vi "sv_Scale Swept Measurements to EU.vi"(4 "response(s) settings.response":T4(array[cluster]) {"channel info"."pregain" format="%.2f"; "channel info"."weighting filter" items=["Linear", "A-weighting", "B-weighting", "C-weighting", "ITU-R 468-4", "Dolby", "CCITT", "C-message", "Wb", "Wc", "Wd", "We", "Wf", "Wh", "Wj", "Wk", "Wm", "AES17 20 kHz lowpass", "AES17 40 kHz lowpass", "AES17 20 kHz highpass", "AES17 40 kHz highpass"]; "channel info"."dB reference" format="%^.1e"; "channel info"."engineering units" items=["custom..."=0, "V"=1, "A"=21, "C"=30, "pC"=31, "s"=32, "-"=29, "Pa"=2, "N"=20, "g"=3, "m/s^2"=4, "m/s"=5, "m"=6, "mm/s"=12, "mm"=13, "micron/s"=14, "micron"=15, "in/s^2"=7, "in/s"=8, "in"=9, "mil/s"=10, "mil"=11, "rad/s^2"=16, "rad/s"=17, "rad"=18, "deg/s^2"=26, "deg/s"=27, "deg"=28, "RPM"=22, "cycle/s^2"=23, "Hz"=24, "cycle"=25, "strain"=19]; "channel info"."sensor sensitivity" format="%#_5f"}, 6 "stimulus settings.stimulus":T5(array[cluster]) {"channel info"."pregain" format="%.2f"; "channel info"."weighting filter" items=["Linear", "A-weighting", "B-weighting", "C-weighting", "ITU-R 468-4", "Dolby", "CCITT", "C-message", "Wb", "Wc", "Wd", "We", "Wf", "Wh", "Wj", "Wk", "Wm", "AES17 20 kHz lowpass", "AES17 40 kHz lowpass", "AES17 20 kHz highpass", "AES17 40 kHz highpass"]; "channel info"."dB reference" format="%^.1e"; "channel info"."engineering units" items=["custom..."=0, "V"=1, "A"=21, "C"=30, "pC"=31, "s"=32, "-"=29, "Pa"=2, "N"=20, "g"=3, "m/s^2"=4, "m/s"=5, "m"=6, "mm/s"=12, "mm"=13, "micron/s"=14, "micron"=15, "in/s^2"=7, "in/s"=8, "in"=9, "mil/s"=10, "mil"=11, "rad/s^2"=16, "rad/s"=17, "rad"=18, "deg/s^2"=26, "deg/s"=27, "deg"=28, "RPM"=22, "cycle/s^2"=23, "Hz"=24, "cycle"=25, "strain"=19]; "channel info"."sensor sensitivity" format="%#_5f"}, 7 "unscaled response magnitude in":dbl format="%.2f", 8 "unscaled measurements":T6 {"harmonic components [ratio]" format="%.2f"; "THD [ratio]" format="%.2f"; "FRF Measurements"."Im [response]" format="%.2f"; "FRF Measurements"."Re [response]" format="%.2f"; "FRF Measurements"."Im [stimulus]" format="%.2f"; "FRF Measurements"."Re [stimulus]" format="%.2f"; "RMS response" format="%.2f"; "RMS stimulus" format="%.2f"}) -> (0 "scaled measurements":T6 {"harmonic components [ratio]" format="%.2f"; "THD [ratio]" format="%.2f"; "FRF Measurements"."Im [response]" format="%.2f"; "FRF Measurements"."Re [response]" format="%.2f"; "FRF Measurements"."Im [stimulus]" format="%.2f"; "FRF Measurements"."Re [stimulus]" format="%.2f"; "RMS response" format="%.2f"; "RMS stimulus" format="%.2f"}, 5 "unscaled response magnitude out":dbl format="%.2f")   [LabVIEW 2017, in "SoundVib_SweptSine.lvlib"]
uses:
  <vilib>/addons/Sound and Vibration/svt_Swept Sine/SoundVib_SweptSine.lvlib
  <vilib>/addons/_NISVFA/_Shared subVIs/Controls/svc_Channel Info.ctl
  <vilib>/addons/_NISVFA/_Shared subVIs/Controls/svc_Engineering Units Text Ring.ctl
  <vilib>/addons/_NISVFA/_Shared subVIs/Controls/svc_Weighting Filter Text Ring.ctl
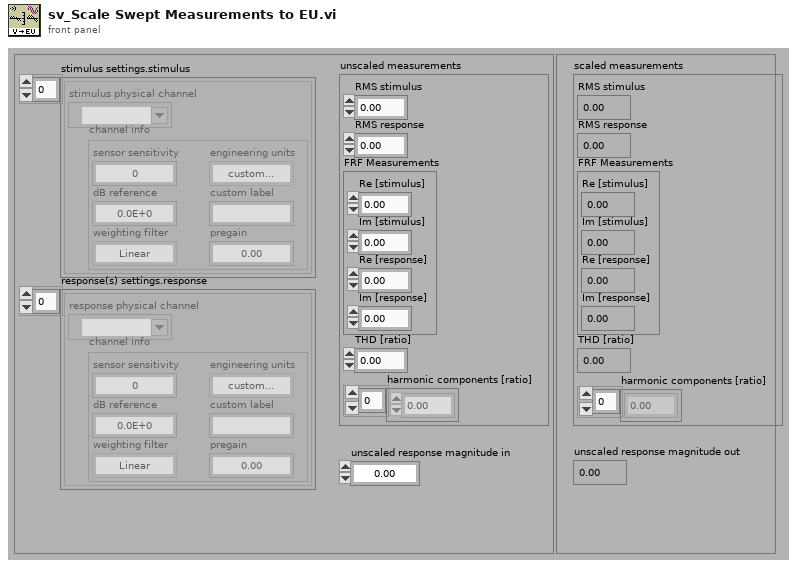
[diagram p1: front panel]
types:
  T1 = typedef "svc_Channel Info.ctl" = cluster{"sensor sensitivity":dbl, "engineering units":T2, "dB reference":dbl, "custom label":string, "weighting filter":T3, "pregain":dbl}
  T2 = typedef "svc_Engineering Units Text Ring.ctl" = u16
  T3 = typedef "svc_Weighting Filter Text Ring.ctl" = u16
  T4 = cluster{"response physical channel":tag, "channel info":T1}[]
  T5 = cluster{"stimulus physical channel":tag, "channel info":T1}[]
  T6 = cluster{"RMS stimulus":dbl, "RMS response":dbl, "FRF Measurements":cluster{"Re [stimulus]":dbl, "Im [stimulus]":dbl, "Re [response]":dbl, "Im [response]":dbl}, "THD [ratio]":dbl, "harmonic components [ratio]":dbl[]}
  T7 = cluster{"Re [stimulus]":dbl, "Im [stimulus]":dbl, "Re [response]":dbl, "Im [response]":dbl}
  T8 = cluster{"stimulus physical channel":tag, "channel info":T1}
  T9 = cluster{"response physical channel":tag, "channel info":T1}
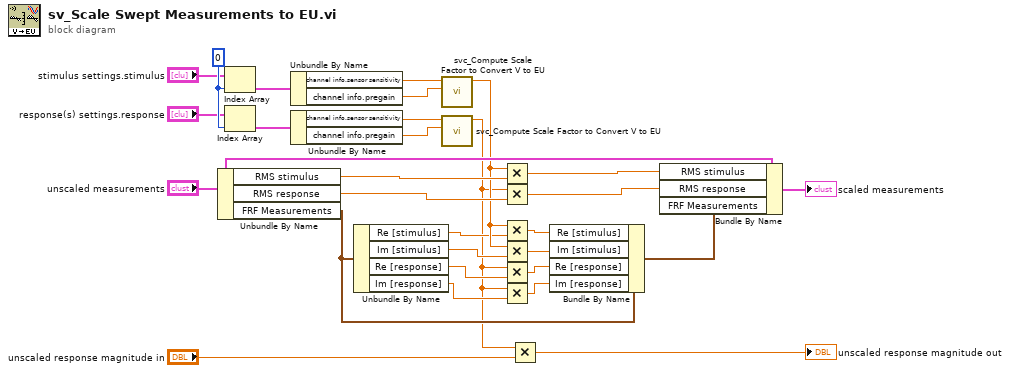
[diagram p0: block diagram]
diagram:
  w10 = 0 ("index")
  n1 = Unbundle By Name("unscaled measurements") -> ("RMS stimulus"=w17:dbl, "RMS response"=w16:dbl, "FRF Measurements"=w21:T7)
  n2 = Index Array(array="stimulus settings.stimulus", index=w10) -> (element=w18:T8)
  n3 = Index Array(array="response(s) settings.response", index=w10) -> (element=w19:T9)
  n4 = Unbundle By Name(w18) -> ("channel info.sensor sensitivity"=w4:dbl, "channel info.pregain"=w3:dbl)
  n5 = Unbundle By Name(w19) -> ("channel info.sensor sensitivity"=w2:dbl, "channel info.pregain"=w1:dbl)
  n6 = Unbundle By Name(w21) -> ("Re [stimulus]"=w14:dbl, "Im [stimulus]"=w13:dbl, "Re [response]"=w12:dbl, "Im [response]"=w11:dbl)
  n7 = call <vilib>:"svc_Compute Scale Factor to Convert V to EU.vi"("pregain [dB]"=w3, "sensor sensitivity [mV/EU]"=w4) -> ("EU scale factor [EU/V]"=w15:dbl)  [unwired: 9 in]
  n8 = call <vilib>:"svc_Compute Scale Factor to Convert V to EU.vi"("pregain [dB]"=w1, "sensor sensitivity [mV/EU]"=w2) -> ("EU scale factor [EU/V]"=w7:dbl)  [unwired: 9 in]
  n9 = Multiply(x=w15, y=w17) -> (x*y=w26:dbl)
  n10 = Multiply(x=w7, y=w16) -> (x*y=w27:dbl)
  n11 = Multiply(x=w15, y=w14) -> (x*y=w22:dbl)
  n12 = Multiply(x=w15, y=w13) -> (x*y=w23:dbl)
  n13 = Multiply(x=w7, y=w12) -> (x*y=w24:dbl)
  n14 = Multiply(x=w7, y=w11) -> (x*y=w25:dbl)
  n15 = Multiply(x=w7, y="unscaled response magnitude in") -> (x*y=→"unscaled response magnitude out":dbl)
  n16 = Bundle By Name(cluster=w21, "Re [stimulus]"=w22, "Im [stimulus]"=w23, "Re [response]"=w24, "Im [response]"=w25) -> (w28:T7)
  n17 = Bundle By Name(cluster="unscaled measurements", "RMS stimulus"=w26, "RMS response"=w27, "FRF Measurements"=w28) -> (→"scaled measurements":T6)
